vi "Tracepoint_SendDataError.vi"(8 "error in (no error)":errorcluster, 9 "message":string, 10 "error code":i32, 11 "Qbus":refnum<class "Qbus.lvclass">) -> (0 "error out":errorcluster)   [LabVIEW 2017, in "FileManager.lvlib"]
uses:
  <vilib>/addons/InsightCM/Devices/Shared/Common/FileManager/FileManager.lvlib
  <vilib>/addons/Qbus/Qbus.lvclass
  <vilib>/addons/TraceLogger/TraceLogger.lvlib
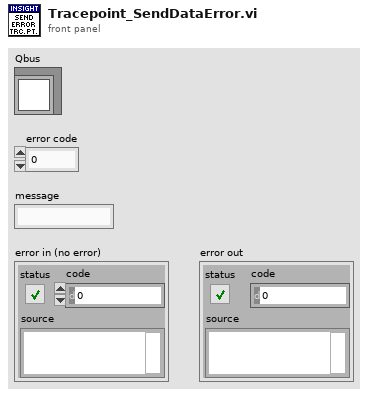
[diagram p1: front panel]
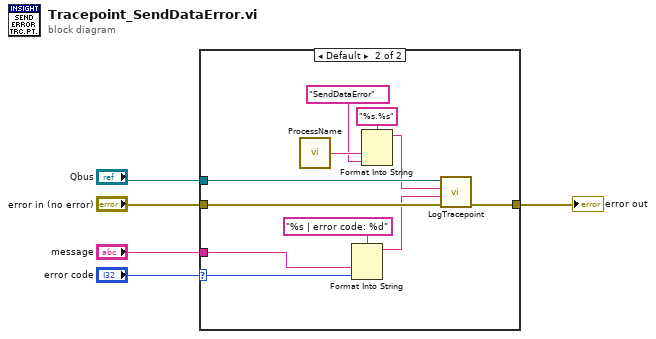
[diagram p0: block diagram]
diagram:
  n1 = case shown="Default" "error code" {
    selector: "error code" -> [_ w7]
    tunnel: "message" -> [_ w17]
    tunnel: [w6 w15] -> w4
    tunnel: "error in (no error)" -> [w6 w14]
    tunnel: "Qbus" -> [_ w13]
    frame 0 {
    }
    frame Default {
      n2 = call <vilib>:"ProcessName.vi"() -> ("process name"=w11:string)  [unwired: 5 in]
      n3 = Format Into String(format string="%s | error code: %d", w17, w7) -> (resulting string=w12:string)  [unwired: 2 in, 1 out]
      n4 = Format Into String(format string="%s.%s", w11, "SendDataError" ("tracepoint")) -> (resulting string=w8:string)  [unwired: 2 in, 1 out]
      n5 = call <vilib>:"LogTracepoint.vi"("error in (no error)"=w14, "log string"=w12, "tracepoint"=w8, "qbus in"=w13) -> ("error out"=w15:errorcluster)  [unwired: 6 in, 1 out]
    }
  }
  "error out" <- w4
